vi "vscan.vi"(3 "Draw":enum16{"I(Ewe)", "Ewe(t)", "I(t)"}(ring)=enum."Ewe(t)", 6 "DLLPath":path, 7 "Essential?":bool=TRUE, 8 "error in (no error)":errorcluster, 9 "VSCAN Parameters":T3={"tb"=5e-05, "vs_initial "=TRUE, "Voltage_step"=0.0, "Scans"=[{" vs_initial "=FALSE, "Voltage_step"=0.1, "Scan_Rate"=0.1}, {" vs_initial "=FALSE, "Voltage_step"=-0.2, "Scan_Rate"=0.1}, {" vs_initial "=FALSE, "Voltage_step"=0.0, "Scan_Rate"=0.1}], "Scan_number"=2, "N_Cycles"=0, "Record_every_dE"=0.01, "Begin_measuring_I"=0.5, "End_measuring_I"=0.75, "I_Range"=12, "E_Range"=3, "Bandwidth"=5, "em"=1, "ce"=0} {"tb" min=5e-05 max=1 format="%^_3e"; "ce" items=["Standard", "CE to ground"]; "End_measuring_I" min=0 max=1 format="%.2f"; "Begin_measuring_I" min=0 max=1 format="%.2f"; "Voltage_step" min=-10 max=10 format="%^_3e"; "N_Cycles" min=0 max=1000000; "Scan_number" min=0 max=98; "Scans"."Scan_Rate" min=1e-05 max=10 format="%^_3e"; "Scans"."Voltage_step" format="%^_3e"; "E_Range" items=["±2.5V", "±5V", "±10V", "Auto"]; "Bandwidth" items=["1"=1, "2"=2, "3"=3, "4"=4, "5"=5, "6"=6, "7"=7, "8"=8, "9"=9]; "Record_every_dE" format="%^_3e"; "I_Range" items=["1pA", "1nA", "10nA", "100nA", "1µA", "10µA", "100µA", "1mA", "10mA", "100mA", "1A", "Booster", "Auto"]}, 10 "Channel":u8(ring) items=["1", "2", "3", "4", "5", "6", "7", "8", "9", "10", "11", "12", "13", "14", "15", "16"], 11 "IP adress":string="192.109.209.229") -> (0 "error out":errorcluster, 1 "XY Graph":cluster{"Data 101":sgl[], "Data 101":sgl[]}(graph)={"Data 101"=[8e-05, 0.1006, 0.20111999, 0.30164, 0.40219998, 0.50272, 0.60324, 0.70375997, 0.80428, 0.90484, 1.002, 1.10252, 1.20304, 1.30356, 1.40412, 1.50464, 1.60516, 1.70568, 1.8061999, 1.90676, 2.0072799, 2.1078, 2.20832, 2.3088799, 2.4094, 2.50992, 2.61044, 2.711, 2.8115199, 2.91204, 3.01256, 3.1131198, 3.21364, 3.3141599, 3.41468, 3.5152, 3.6157598, 3.71628, 3.8167999, 3.91732, 4.00108, 4.1015997, 4.20212, 4.30264, 4.4031997, 4.50372, 4.60424, 4.70476, 4.8052797, 4.90584, 5.00636, 5.1068797, 5.2074, 5.30796, 5.4084797, 5.509, 5.60952, 5.7100797, 5.8106, 5.91112], "Data 101"=[4.2835555e-07, 2.1494968e-06, 4.146294e-06, 6.138965e-06, 8.133681e-06, 1.0123058e-05, 1.2087297e-05, 1.4083101e-05, 1.6065378e-05, 1.80591e-05, 1.9984154e-05, 1.7937375e-05, 1.595267e-05, 1.3964497e-05, 1.197563e-05, 9.982255e-06, 7.9902675e-06, 6.0027883e-06, 3.9787647e-06, 1.9855738e-06, -3.2822256e-09, -1.9828094e-06, -3.9722895e-06, -5.9632257e-06, -7.95541e-06, -9.9489125e-06, -1.1902557e-05, -1.389385e-05, -1.5878555e-05, -1.7874703e-05, -1.9867039e-05, -2.1852784e-05, -2.3842693e-05, -2.583641e-05, -2.7823196e-05, -2.9813451e-05, -3.180405e-05, -3.3791526e-05, -3.5780395e-05, -3.777169e-05, -3.9435956e-05, -3.7391255e-05, -3.539476e-05, -3.3405893e-05, -3.1415642e-05, -2.9424347e-05, -2.7433402e-05, -2.5453895e-05, -2.3455323e-05, -2.1465068e-05, -1.9473428e-05, -1.7484906e-05, -1.5494306e-05, -1.3505094e-05, -1.1516228e-05, -9.523894e-06, -7.5357216e-06, -5.542347e-06, -3.5301439e-06, -1.543508e-06]}, 2 "output essential":T2, 4 "output premium":T1, 5 "Exit 2":bool=TRUE)   [LabVIEW 2022 SP3]
doc: "The VSCAN ( Potentiodynamic Technique) consists of scanning linearly the potential of a stationary working electrode with different scan rates.\nIn general, in this VI, the first thing to do is to start by establishing the connection with the instrument defined by its IP adress, then load the firmware in the channel selected, get the information on the plugged channels, load protocol on a channel, start/stop the protocol, retreive data and draw the graph."
uses:
  Library/EClib Functions/VSCANParameters.ctl
  Library/EClib Functions/Parameters.ctl
  Library/EClib Functions/EClib functions.lvlib
panel:
  out "cycle index":i32[](array[numeric])
  in  "Display Parameters?":bool caption="Display Parameters"
  out "DllPath":path caption="DLL Path"
  out "LibVersion":string caption="DLL Version"
  out "Device Code":i32=12
  out "Number of points":i32=60
  out "Data 124":sgl[][](array[numeric])=[[8e-05, -0.00015008324, 4.2835555e-07, 0.0013634439, 1.0], [0.1006, 0.009902848, 2.1494968e-06, 0.010471455, 1.0], [0.20111999, 0.019955778, 4.146294e-06, 0.02059764, 1.0], [0.30164, 0.030008709, 6.138965e-06, 0.030609425, 1.0], [0.40219998, 0.04006164, 8.133681e-06, 0.04071481, 1.0], [0.50272, 0.050114572, 1.0123058e-05, 0.05077513, 1.0], [0.60324, 0.060167503, 1.2087297e-05, 0.06075918, 1.0], [0.70375997, 0.07022043, 1.4083101e-05, 0.07082297, 1.0], [0.80428, 0.08027337, 1.6065378e-05, 0.080852084, 1.0], [0.90484, 0.090326294, 1.80591e-05, 0.090902, 1.0], [1.002, 0.10004413, 1.9984154e-05, 0.100629516, 1.0], [1.10252, 0.0899912, 1.7937375e-05, 0.09124173, 1.0], [1.20304, 0.07993827, 1.595267e-05, 0.08120915, 1.0], [1.30356, 0.069885336, 1.3964497e-05, 0.0711627, 1.0], [1.40412, 0.059832405, 1.197563e-05, 0.06106771, 1.0], [1.50464, 0.049779475, 9.982255e-06, 0.051007397, 1.0], [1.60516, 0.039726544, 7.9902675e-06, 0.040967878, 1.0], [1.70568, 0.029673612, 6.0027883e-06, 0.030924892, 1.0], [1.8061999, 0.019620681, 3.9787647e-06, 0.020868042, 1.0], [1.90676, 0.009567751, 1.9855738e-06, 0.010804256, 1.0], [2.0072799, -0.00048518094, -3.2822256e-09, 0.0006746042, 1.0], [2.1078, -0.010538111, -1.9828094e-06, -0.009257445, 1.0], [2.20832, -0.020591041, -3.9722895e-06, -0.019307364, 1.0], [2.3088799, -0.030643972, -5.9632257e-06, -0.029412746, 1.0], [2.4094, -0.0406969, -7.95541e-06, -0.039452266, 1.0], [2.50992, -0.050749835, -9.9489125e-06, -0.049533386, 1.0], [2.61044, -0.060802765, -1.1902557e-05, -0.059479296, 1.0], [2.711, -0.07085569, -1.389385e-05, -0.06955695, 1.0], [2.8115199, -0.08090863, -1.5878555e-05, -0.07963461, 1.0], [2.91204, -0.09096155, -1.7874703e-05, -0.08969492, 1.0], [3.01256, -0.10101449, -1.9867039e-05, -0.09973444, 1.0], [3.1131198, -0.111067414, -2.1852784e-05, -0.1098225, 1.0], [3.21364, -0.12112035, -2.3842693e-05, -0.119851604, 1.0], [3.3141599, -0.13117327, -2.583641e-05, -0.12988071, 1.0], [3.41468, -0.1412262, -2.7823196e-05, -0.13995838, 1.0], [3.5152, -0.15127914, -2.9813451e-05, -0.15000136, 1.0], [3.6157598, -0.16133207, -3.180405e-05, -0.16006514, 1.0], [3.71628, -0.17138499, -3.3791526e-05, -0.1701324, 1.0], [3.8167999, -0.18143792, -3.5780395e-05, -0.18019964, 1.0], [3.91732, -0.19149086, -3.777169e-05, -0.19023915, 1.0], [4.00108, -0.1998683, -3.9435956e-05, -0.19861813, 1.0], [4.1015997, -0.18981537, -3.7391255e-05, -0.1892373, 1.0], [4.20212, -0.17976244, -3.539476e-05, -0.17914924, 1.0], [4.30264, -0.1697095, -3.3405893e-05, -0.16911319, 1.0], [4.4031997, -0.15965658, -3.1415642e-05, -0.15908061, 1.0], [4.50372, -0.14960365, -2.9424347e-05, -0.14899254, 1.0], [4.60424, -0.13955072, -2.7433402e-05, -0.13895303, 1.0], [4.70476, -0.12949778, -2.5453895e-05, -0.12891698, 1.0], [4.8052797, -0.119444855, -2.3455323e-05, -0.11883587, 1.0], [4.90584, -0.10939193, -2.1465068e-05, -0.10876862, 1.0], [5.00636, -0.09933899, -1.9473428e-05, -0.098690964, 1.0], [5.1068797, -0.08928607, -1.7484906e-05, -0.088686116, 1.0], [5.2074, -0.07923313, -1.5494306e-05, -0.07859806, 1.0], [5.30796, -0.069180205, -1.3505094e-05, -0.06854121, 1.0], [5.4084797, -0.059127275, -1.1516228e-05, -0.05848783, 1.0], [5.509, -0.049074344, -9.523894e-06, -0.048455246, 1.0], [5.60952, -0.039021414, -7.5357216e-06, -0.038367193, 1.0], [5.7100797, -0.028968483, -5.542347e-06, -0.028327677, 1.0], [5.8106, -0.018915553, -3.5301439e-06, -0.018236158, 1.0], [5.91112, -0.008862623, -1.543508e-06, -0.008182773, 1.0]] format="%.2f"
  in  "stop":bool
  in  "Exit":bool
  in  "Start":bool
  # "Instructions:\nBefore running the VI you must type a valid IP adress that corresponds to the instrument.Then press the Run button to execute this VI.\nWhile this VI is running, choose the available channel, enter the VSCAN parameters or keep the default values, then press the button start to begin the experience.\nChoose the waveform to draw (Ewe(t) or I(t) or I(Ewe) or Ec(t). You can stop the measure if you press the stop button and exit the execution if you press the exit button."
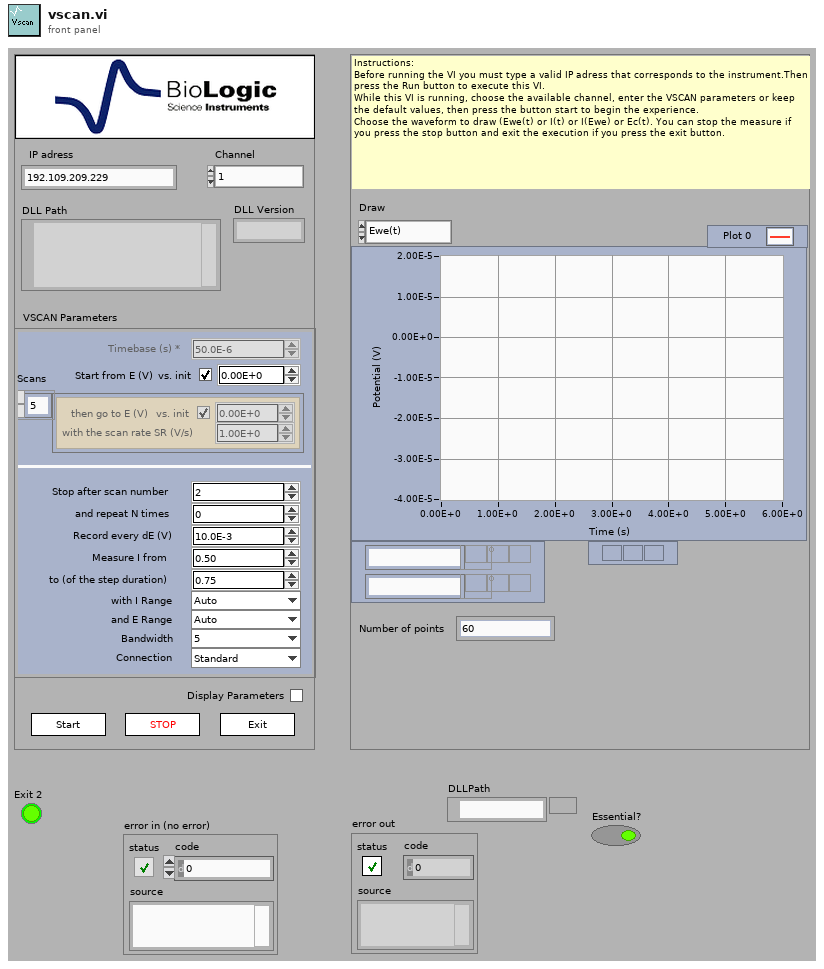
[diagram p1: front panel]
types:
  T1 = cluster{"Data 124":sgl[], "Data 124":sgl[], "Data 124":sgl[], "cycle index":u32[]}
  T2 = cluster{"Data 124":sgl[], "Data 124":sgl[], "Data 124":sgl[], "Data 124":sgl[], "cycle index":i32[]}
  T3 = typedef "EClib functions.lvlib/VSCANParameters.ctl" = cluster{"tb":sgl, "vs_initial ":bool, "Voltage_step":sgl, "Scans":cluster{" vs_initial ":bool, "Voltage_step":sgl, "Scan_Rate":sgl}[], "Scan_number":i32, "N_Cycles":i32, "Record_every_dE":sgl, "Begin_measuring_I":sgl, "End_measuring_I":sgl, "I_Range":u16, "E_Range":u16, "Bandwidth":u16, "em":u16, "ce":u16}
  T4 = cluster{"LibVersion":string, "StringLength":u32, "DllPath":path}
  T5 = cluster{"Channel":i32, "BoardVersion":i32, "BoardSerialCode":i32, "FirmwareCode":i32, "FirmwareVersion":i32, "XilinxVersion":i32, "AmpCode":i32, "NbAmp":i32, "LcBoard":i32, "Zboard":i32, "MuxBoard":i32, "GPRAboard":i32, "MemSize":i32, "MemFilled":i32, "state":i32, "MaxIRange":i32, "MinIRange":i32, "MaxBandwidth":i32, "NbOfTechniques":i32}
  T6 = typedef "EClib functions.lvlib/Parameters.ctl" = enum16{"CA", "CASG", "CP", "GEIS", "ISCAN", "OCV", "PEIS", "SCCX", "SGEIS", "SPEIS", "VSCAN", "MP"}
  T7 = typedef "EClib functions.lvlib/TechniqueParameters.ctl" = cluster{"String Label":string, "Type":i32, "Valeur":i32, "Index":i32}
  T8 = cluster{"string before end tag":string, i32, i32, i32}[]
  T9 = cluster{"IRQskipped":i32, "NbRaws":i32, "NbCols":i32, "Technique Index":i32, "TechniqueID":i32, "PrcessIndex":i32, "loop":i32, "StartTime":dbl, "MuxPad":i32}
  T10 = cluster{"State":i32, "MemFilled":i32, "TimeBase":sgl, " Ewe":sgl, " EweRangeMin":sgl, " EweRangeMax":sgl, "Ece":sgl, "EceRangeMin":sgl, "EceRangeMax":sgl, "Eoverflow":i32, "I":sgl, "IRange":i32, "Ioverflow":i32, "ElapsedTime":sgl, "Freq":sgl, "Rcomp":sgl, "Saturation":sgl, "OptErr":i32, "OptPos":i32}
  T11 = cluster{"Data 124":sgl[], "Data 124":sgl[], "Data 124":sgl[], "cycle index":i32[]}
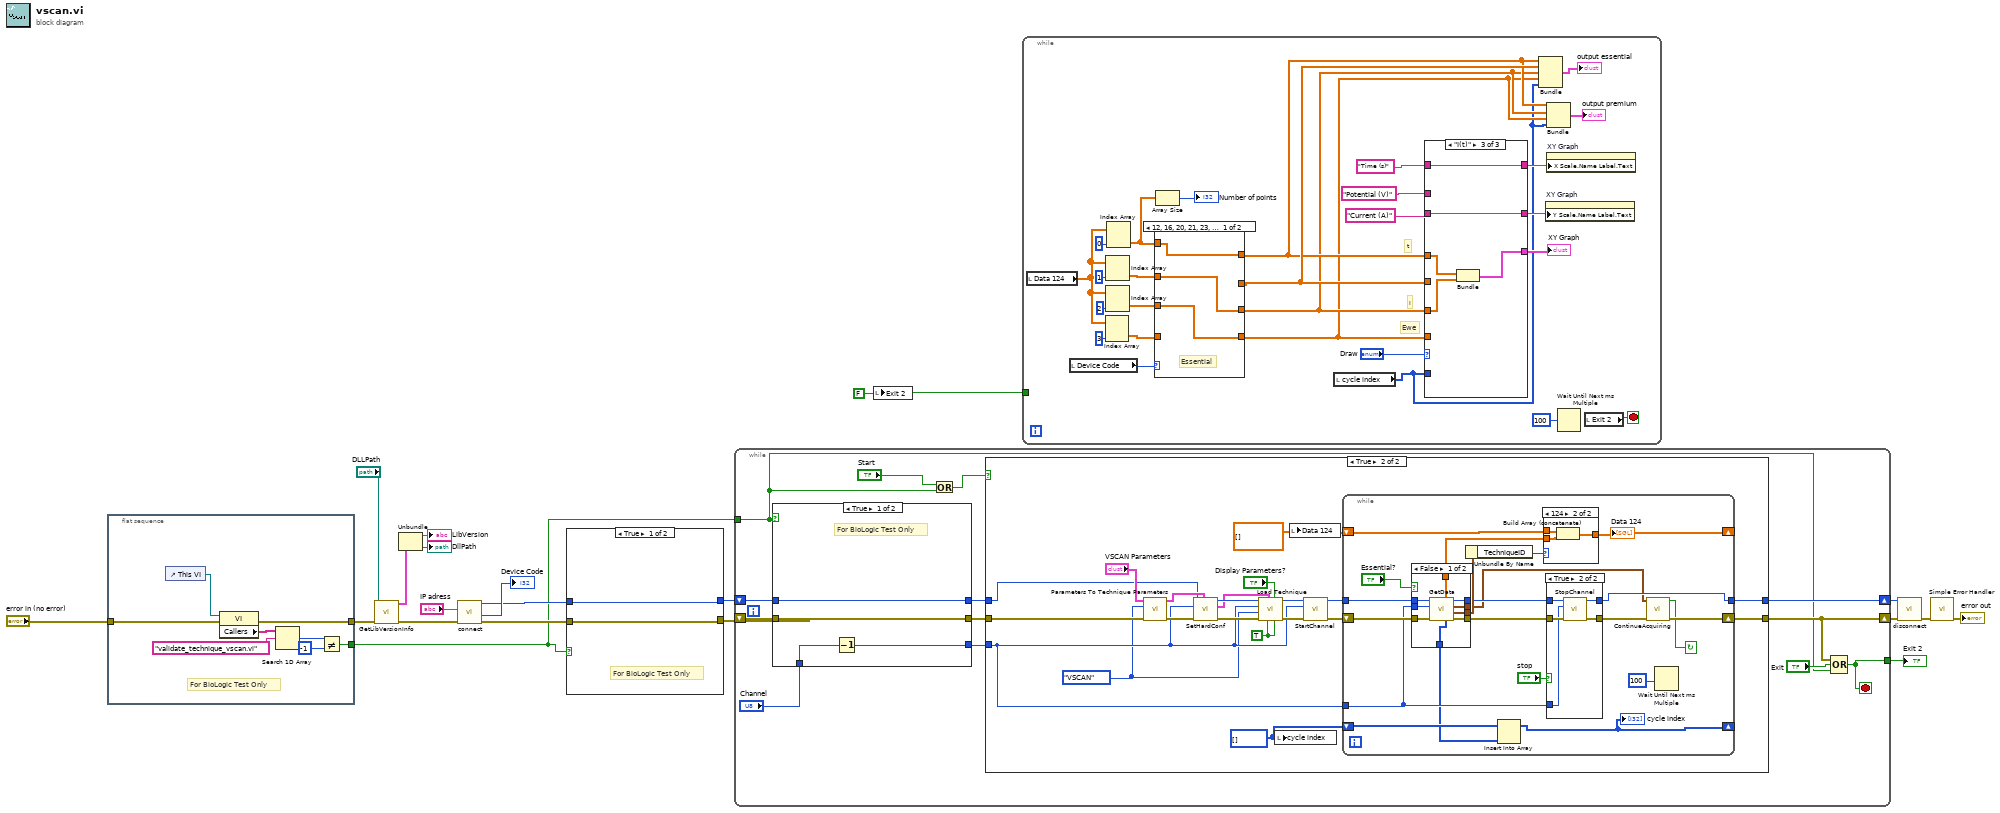
[diagram p0: block diagram]
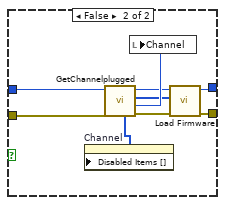
[diagram p2: hidden frame]
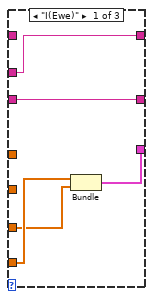
[diagram p3: hidden frame]
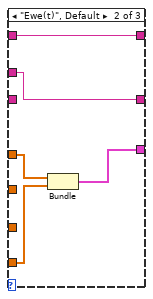
[diagram p4: hidden frame]
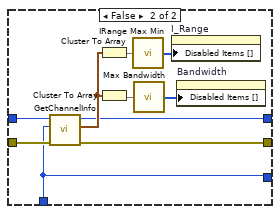
[diagram p6: hidden frame]
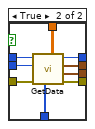
[diagram p8: hidden frame]
diagram:
  w19 = FALSE ("Exit 2")
  n1 = flat-sequence {
    tunnel: "error in (no error)" -> [w27]
    tunnel: [w26] -> w5
    tunnel: [w21] -> w3
    frame #0 {
      # "For BioLogic Test Only"
      n2 = control-ref of="This VI"() -> (w28:refnum<vi>)
      n3 = property class="VI"(reference=w28, error in=w27) -> (error out=w26:errorcluster, "Callers"=w25:string[])  [unwired: 1 out]
      n4 = Search 1D Array(1D array=w25, element="validate_technique_vscan.vi") -> (index of element=w23:i32)  [unwired: 1 in]
      n5 = Not Equal?(x=w23, y=-1) -> (x != y?=w21:bool)
    }
  }
  n6 = call "GetLibVersionInfo.vi"("error in (no error)"=w5, "DLLPath"="DLLPath") -> ("error out"=w9:errorcluster, "LibInfo"=w12:T4)  [unwired: 8 in]
  n7 = Unbundle(w12) -> ("LibVersion"=→"LibVersion":string, "DllPath"=→"DllPath":path)  [unwired: 1 out]
  n8 = call "connect.vi"("error in (no error)"=w9, "IP"="IP adress") -> ("error out"=w16:errorcluster, "Device Code"=→"Device Code":i32, "ID Out"=w7:i32)  [unwired: 5 in, 2 out]
  n9 = case shown="True" w3 {
    tunnel: w16 -> [w30 w37]
    tunnel: [w30 w33] -> w15
    tunnel: [w29 w31] -> w6
    tunnel: w7 -> [w29 w32]
    frame True {
      # "For BioLogic Test Only"
    }
    frame False {
      n10 = call "GetChannelplugged.vi"("error in (no error)"=w37, "ID In"=w32) -> ("error out"=w36:errorcluster, "FirstPluggedChannel"=w38:u8, "PluggedChannels"=w34:u8[], "DisabledChannels"=w35:i32[])  [unwired: 5 in, 1 out]
      n11 = property on="Channel" class="Ring (strict)"("Disabled Items []"=w35) -> ()  [unwired: 2 in, 2 out]
      n12 = local write "Channel"(w38) -> ()
      n13 = call "Load Firmware.vi"("error in (no error)"=w36, "Channels"=w34, "ID In"=w32) -> ("error out"=w33:errorcluster, "ID Out"=w31:i32)  [unwired: 6 in, 1 out]
    }
  }
  n14 = while {
    shift-right: [w46] -> w14
    shift-left: w15 -> [w50]
    tunnel: [w44] -> w20
    shift-right: [w47] -> w17
    shift-left: w6 -> [w51]
    tunnel: w3 -> [w39]
    stop <- w44 stop-if-true
    n15 = case shown="True" w39 {
      tunnel: w51 -> [w53 w61]
      tunnel: w50 -> [w52 w60]
      tunnel: [w52 w59] -> w49
      tunnel: "Channel" -> [w55 w56]
      tunnel: [w53 w57] -> w48
      tunnel: [w54 w56] -> w42
      frame True {
        # "For BioLogic Test Only"
        n16 = Decrement(x=w55) -> (x-1=w54:u8)
      }
      frame False {
        n17 = call "GetChannelInfo.vi"("error in (no error)"=w60, "Channel"=w56, "ID"=w61) -> ("error out"=w59:errorcluster, "Channel information"=w58:T5, "ID Out"=w57:i32)  [unwired: 6 in]
        n18 = Cluster To Array(cluster=w58) -> (array=w65:i32[])
        n19 = Cluster To Array(cluster=w58) -> (array=w64:i32[])
        n20 = call "IRange Max Min.vi"("resources"=w65) -> ("disabled ranges"=w62:i32[])
        n21 = call "Max Bandwidth.vi"("resources"=w64) -> ("disabled ranges"=w63:i32[])
        n22 = property on="I_Range" class="Ring (strict)"("Disabled Items []"=w62) -> ()  [unwired: 2 in, 2 out]
        n23 = property on="Bandwidth" class="Ring (strict)"("Disabled Items []"=w63) -> ()  [unwired: 2 in, 2 out]
      }
    }
    n24 = Or(x="Start", y=w39) -> (x .or. y?=w40:bool)
    n25 = case shown="True" w40 {
      tunnel: w42 -> [_ w70]
      tunnel: [w67 w80] -> w46
      tunnel: w49 -> [w67 w71]
      tunnel: w48 -> [w66 w69]
      tunnel: [w66 w79] -> w47
      frame False {
      }
      frame True {
        w72 = i32[] [] ("cycle index")
        w68 = Parameters."VSCAN" ("Parameters")
        w85 = TRUE ("First Protocol")
        w87 = sgl[][] []
        n26 = call "Parameters To Technique Parameters.vi"("error in (no error)"=w71, "Parameters"=w68, "ParameterIN"="VSCAN Parameters") -> ("error out"=w78:errorcluster, "Params Values"=w74:T7[])  [unwired: 7 in]
        n27 = call "SetHardConf.vi"("Params Values"=w74, "error in (no error)"=w78, "Channel"=w70, "ID In"=w69) -> ("error out"=w77:errorcluster, "Params Values Trimed"=w75:T8, "ID Out"=w76:i32)  [unwired: 5 in]
        n28 = call "Load Technique.vi"("Last Protocol"=w85, "Display Parameters?"="Display Parameters?", "First Protocol"=w85, "TechniqueParameters"=w75, "error in (no error)"=w77, "Parameters"=w68, "Selected Channel"=w70, "ID In"=w76) -> ("error out"=w84:errorcluster, "ID  Out"=w83:i32)  [unwired: 1 in, 1 out]
        n29 = local write "cycle index"(w72) -> ()
        n30 = local write "Data 124"(w87) -> ()
        n31 = call "StartChannel.vi"("error in (no error)"=w84, "Channel"=w70, "ID In"=w83) -> ("error out"=w82:errorcluster, "ID Out"=w81:i32)  [unwired: 7 in]
        n32 = while {
          shift-right: [w95] -> w80
          shift-left: w82 -> [w107]
          shift-right: [w104] -> _
          shift-left: w87 -> [w105]
          tunnel: w70 -> [w97]
          tunnel: w81 -> [w99]
          tunnel: [w96] -> w79
          shift-right: [w90] -> _
          shift-left: w72 -> [w91]
          stop <- w93 continue-if-true
          n33 = case shown="False" "Essential?" {
            tunnel: [w117 w126] -> w108
            tunnel: w107 -> [w116 w125]
            tunnel: [w115 w124] -> w103
            tunnel: [w114 w123] -> w100
            tunnel: w99 -> [w113 w122]
            tunnel: [w112 w121] -> w98
            tunnel: w97 -> [w111 w120]
            tunnel: [w110 w119] -> w92
            tunnel: [w109 w118] -> w89
            frame False {
              n34 = call "GetData.vi"("error in (no error)"=w116, "Channel"=w111, "ID In"=w113) -> ("error out"=w115:errorcluster, "Data information"=w117:T9, "Current values"=w110:T10, "ID Out"=w112:i32, "row2"=w109:u32[], "Data"=w114:dbl[][])  [unwired: 1 in, 2 out]
            }
            frame True {
              n35 = call "GetData.vi"("error in (no error)"=w125, "Channel"=w120, "ID In"=w122) -> ("error out"=w124:errorcluster, "Data information"=w126:T9, "Current values"=w119:T10, "ID Out"=w121:i32, "Data"=w123:dbl[][], "row3"=w118:u32[])  [unwired: 1 in, 2 out]
            }
          }
          n36 = Unbundle By Name(w108) -> ("TechniqueID"=w102:i32)
          n37 = Insert Into Array(array=w91, new element=w89) -> (w90:i32[])  [unwired: 1 in]
          "cycle index" <- w90
          n38 = case shown="124" w102 {
            tunnel: w100 -> [_ w137]
            tunnel: w105 -> [w134 w136]
            tunnel: [w134 w135] -> w104
            frame 0, Default {
            }
            frame 124 {
              n39 = Build Array (concatenate)(w136, w137) -> (w135:dbl[][])
            }
          }
          "Data 124" <- w104
          n40 = case shown="True" "stop" {
            tunnel: [w128 w133] -> w94
            tunnel: w103 -> [w128 w132]
            tunnel: w98 -> [w127 w131]
            tunnel: w97 -> [_ w130]
            tunnel: [w127 w129] -> w96
            frame False {
            }
            frame True {
              n41 = call "StopChannel.vi"("error in (no error)"=w132, "Channel"=w130, "ID In"=w131) -> ("error out"=w133:errorcluster, "ID Out"=w129:i32)  [unwired: 7 in]
            }
          }
          n42 = call "ContinueAcquiring.vi"("error in"=w94, "Current values"=w92) -> ("error out"=w95:errorcluster, "ContinueAcquiring?"=w93:bool)  [unwired: 8 in]
          n43 = Wait Until Next ms Multiple(millisecond multiple=u32 100) -> ()  [unwired: 1 out]
        }
      }
    }
    n44 = Compound Arithmetic op=OR(w46, "Exit", w39) -> (w44:bool)
  }
  "Exit 2" <- w20
  n45 = local write "Exit 2"(w19) -> ()
  n46 = while {
    tunnel: w19 -> [_]
    stop <- w163 stop-if-true
    # "Ewe"
    # "I"
    # "t"
    n47 = local read "Data 124"() -> (w154:sgl[][])
    n48 = local read "Device Code"() -> (w152:i32)
    n49 = Index Array(array=w154, index (col)=3 ("Index")) -> (element=w156:sgl[])  [unwired: 1 in]
    n50 = Index Array(array=w154, index (col)=1 ("Index")) -> (element=w159:sgl[])  [unwired: 1 in]
    n51 = Index Array(array=w154, index (col)=2 ("Index")) -> (element=w157:sgl[])  [unwired: 1 in]
    n52 = Index Array(array=w154, index (col)=0 ("Index")) -> (element=w153:sgl[])  [unwired: 1 in]
    n53 = case shown="12, 16, 20, 21, 23, 27" w152 {
      tunnel: w159 -> [w181 w183]
      tunnel: w157 -> [w180 w185]
      tunnel: w156 -> [_ w184]
      tunnel: w153 -> [w182 w186]
      tunnel: [w182 w186] -> w143
      tunnel: [w181 w185] -> w142
      tunnel: [w180 w184] -> w141
      tunnel: [_ w183] -> w144
      frame 12, 16, 20, 21, 23, 27 {
        # "Essential"
      }
      frame Default {
        # "Premium"
      }
    }
    n54 = Array Size(array=w153) -> (size(s)=→"Number of points":i32)
    n55 = local read "cycle index"() -> (w140:i32[])
    n56 = case shown="\"I(t)\"" "Draw" {
      tunnel: w143 -> [_ w174 w179]
      tunnel: w142 -> [w166 _ w178]
      tunnel: [w165 w170 w175] -> w151
      tunnel: "Potential (V)" ("Y Scale.Name Label.Text") -> [w169 w173 _]
      tunnel: "Current (A)" ("Y Scale.Name Label.Text") -> [w168 _ w177]
      tunnel: [w168 w173 w177] -> w150
      tunnel: [w169 w172 w176] -> w149
      tunnel: "Time (s)" ("Y Scale.Name Label.Text") -> [_ w172 w176]
      tunnel: w141 -> [w167 w171 _]
      tunnel: w144 -> [_ _ _]
      tunnel: w140 -> [_ _ _]
      frame "I(Ewe)" {
        n57 = Bundle("Data 124"=w167, "Data 124"=w166) -> (w165:cluster{"Data 124":sgl[], "Data 124":sgl[]})  [unwired: 1 in]
      }
      frame "Ewe(t)", Default {
        n58 = Bundle("Data 124"=w174, "Data 124"=w171) -> (w170:cluster{"Data 124":sgl[], "Data 124":sgl[]})  [unwired: 1 in]
      }
      frame "I(t)" {
        n59 = Bundle("Data 124"=w179, "Data 124"=w178) -> (w175:cluster{"Data 124":sgl[], "Data 124":sgl[]})  [unwired: 1 in]
      }
    }
    "XY Graph" <- w151
    n60 = Bundle("Data 124"=w143, "Data 124"=w144, "Data 124"=w142, "Data 124"=w141, "cycle index"=w140) -> (→"output essential":T2)  [unwired: 1 in]
    n61 = property on="XY Graph" class="XYGraph (strict)"("Y Scale.Name Label.Text"=w150) -> ()  [unwired: 2 in, 2 out]
    n62 = Bundle("Data 124"=w143, "Data 124"=w142, "Data 124"=w141, "cycle index"=w140) -> (→"output premium":T11)  [unwired: 1 in]
    n63 = property on="XY Graph" class="XYGraph (strict)"("X Scale.Name Label.Text"=w149) -> ()  [unwired: 2 in, 2 out]
    n64 = Wait Until Next ms Multiple(millisecond multiple=u32 100) -> ()  [unwired: 1 out]
    n65 = local read "Exit 2"() -> (w163:bool)
  }
  n66 = call "disconnect.vi"("error in (no error)"=w14, "ID In"=w17) -> ("error out"=w13:errorcluster)  [unwired: 9 in]
  n67 = call <vilib>:"Simple Error Handler.vi"("error in (no error)"=w13) -> ("error out"=→"error out":errorcluster)  [unwired: 4 in, 4 out]
